vi "Test Model Fit.vi"() -> ()   [LabVIEW 2015]
uses:
  Typedefs/PSTR-Fit Parameters.ctl
  Utility VIs/Math VIs/LinSpace (x0-dx-npts).vi
  <vilib>/Analysis/NI_AALBase.lvlib
panel:
  out "Fit":T1
  out "XY Graph":cluster{"t":dbl[], "y":dbl[]}[](graph)
  in  "Latency (ms)":dbl=5.0
  in  "Duration (ms)":dbl=300.0
  in  "Fs (Hz)":dbl=100000.0
  in  "Delay (ms)":dbl=100.0
  in  "Parameters":T1={"Ar"=4.0, "Tr"=5.0, "Ast"=0.5, "Tst"=20.0, "Ass"=0.4}
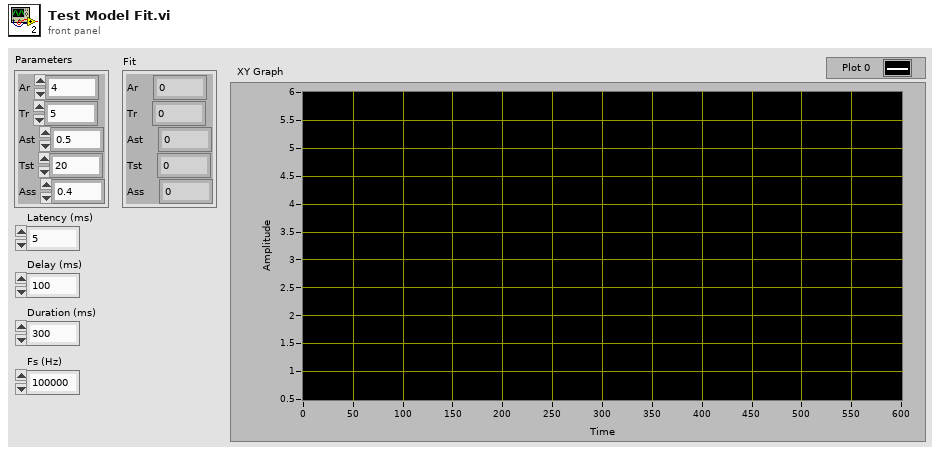
[diagram p1: front panel]
types:
  T1 = typedef "PSTR-Fit Parameters.ctl" = cluster{"Ar":dbl, "Tr":dbl, "Ast":dbl, "Tst":dbl, "Ass":dbl}
  T2 = typedef "PSTR-Model Fit.ctl" = cluster{"Parameters":T1, "t":dbl[], "y":dbl[], "R2":dbl}
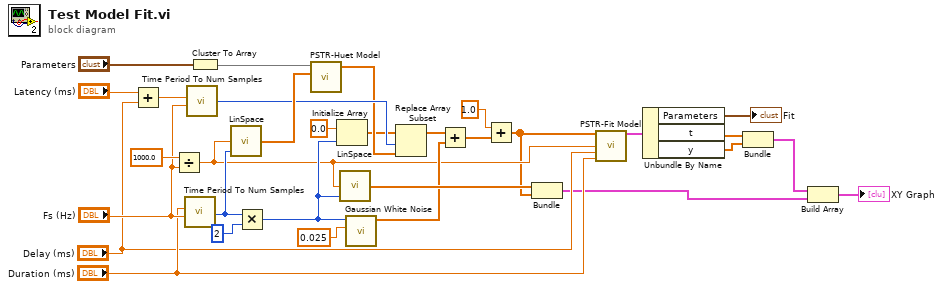
[diagram p0: block diagram]
diagram:
  n1 = Add(x="Latency (ms)", y="Delay (ms)") -> (x+y=w24:dbl)
  n2 = Divide(x=1000.0, y="Fs (Hz)") -> (x/y=w12:dbl)
  n3 = call "Time Period To Num Samples.vi"("Duration (ms)"="Duration (ms)", "Sampling rate (Hz)"="Fs (Hz)") -> ("Samples"=w28:i32)  [unwired: 5 in]
  n4 = call "Time Period To Num Samples.vi"("Duration (ms)"=w24, "Sampling rate (Hz)"="Fs (Hz)") -> ("Samples"=w21:i32)  [unwired: 5 in]
  n5 = Cluster To Array(cluster="Parameters") -> (array=w30:dbl[])
  n6 = call-poly "LinSpace.vi"("npts"=w28, "dx"=w12) -> ("Array"=w26:dbl[])  [unwired: 2 in, 1 out]
  n7 = Multiply(x=w28, y=2) -> (x*y=w17:i32)
  n8 = call "PSTR-Huet Model.vi"("X"=w26, "a"=w30) -> ("f(X,a)"=w20:dbl[])  [unwired: 2 in, 2 out]
  n9 = Initialize Array(0.0 ("element"), w17) -> (w15:dbl[])
  n10 = call-poly "LinSpace.vi"("npts"=w17, "dx"=w12) -> ("Array"=w22:dbl[])  [unwired: 2 in, 1 out]
  n11 = call <vilib>:"Gaussian White Noise.vi"("standard deviation"=0.025, "samples"=w17) -> ("Gaussian noise pattern"=w14:dbl[])  [unwired: 8 in, 1 out]
  n12 = Replace Array Subset(array=w15, new element=w20, index=w21) -> (w19:dbl[])
  n13 = Add(x=w19, y=w14) -> (x+y=w13:dbl[])
  n14 = Add(x=1.0, y=w13) -> (x+y=w7:dbl[])
  n15 = Bundle("Array"=w22, w7) -> (w1:cluster{"Array":dbl[], dbl[]})  [unwired: 1 in]
  n16 = call "PSTR-Fit Model.vi"("PSTH"=w7, "dt (ms)"=w12, "delay (ms)"="Delay (ms)", "durat (ms)"="Duration (ms)") -> ("Fit"=w9:T2)  [unwired: 11 in]
  n17 = Unbundle By Name(w9) -> ("Parameters"=→"Fit":T1, "t"=w5:dbl[], "y"=w4:dbl[])
  n18 = Bundle("t"=w5, "y"=w4) -> (w3:cluster{"t":dbl[], "y":dbl[]})  [unwired: 1 in]
  n19 = Build Array(w3, w1) -> (→"XY Graph":cluster{"Array":dbl[], "y":dbl[]}[])
